vi "Update Field for Spartan 5.0.vi"(8 "error in (no error)":errorcluster, 10 "Old Field Record":T1={"ixField"=0, "iSequenceOrder"=0, "sxFieldId"="", "sxSequenceId"="", "sDisplayName"="", "sValue"="", "sUnits"="", "nDataType"=enum."timestamp", "nNextItem"=enum."Reset", "fSystem"=FALSE, "fSystemValue"=FALSE, "fRequired"=FALSE, "fSetAtTest"=FALSE, "fTestField"=FALSE, "fDeleted"=FALSE, "fIndexed"=FALSE, "fFreeList"=FALSE}) -> (0 "error out":errorcluster, 2 "New Field Record":T1={"ixField"=0, "iSequenceOrder"=0, "sxFieldId"="", "sxSequenceId"="", "sDisplayName"="", "sValue"="", "sUnits"="", "nDataType"=enum."timestamp", "nNextItem"=enum."Reset", "fSystem"=FALSE, "fSystemValue"=FALSE, "fRequired"=FALSE, "fSetAtTest"=FALSE, "fTestField"=FALSE, "fDeleted"=FALSE, "fIndexed"=FALSE, "fFreeList"=FALSE})   [LabVIEW 2011]
uses:
  Field Record.ctl
  Field DataTypes.ctl
  Field NextItem.ctl
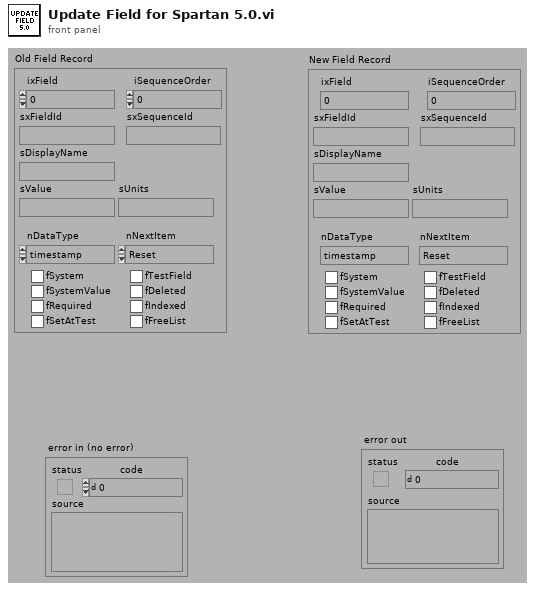
[diagram p1: front panel]
types:
  T1 = typedef "Field Record.ctl" = cluster{"ixField":i32, "iSequenceOrder":i32, "sxFieldId":string, "sxSequenceId":string, "sDisplayName":string, "sValue":string, "sUnits":string, "nDataType":T2, "nNextItem":T3, "fSystem":bool, "fSystemValue":bool, "fRequired":bool, "fSetAtTest":bool, "fTestField":bool, "fDeleted":bool, "fIndexed":bool, "fFreeList":bool}
  T2 = typedef "Field DataTypes.ctl" = enum32{"text", "numeric", "list", "timestamp", "boolean"}
  T3 = typedef "Field NextItem.ctl" = enum32{"Reset", "Retain", "Auto-Increment"}
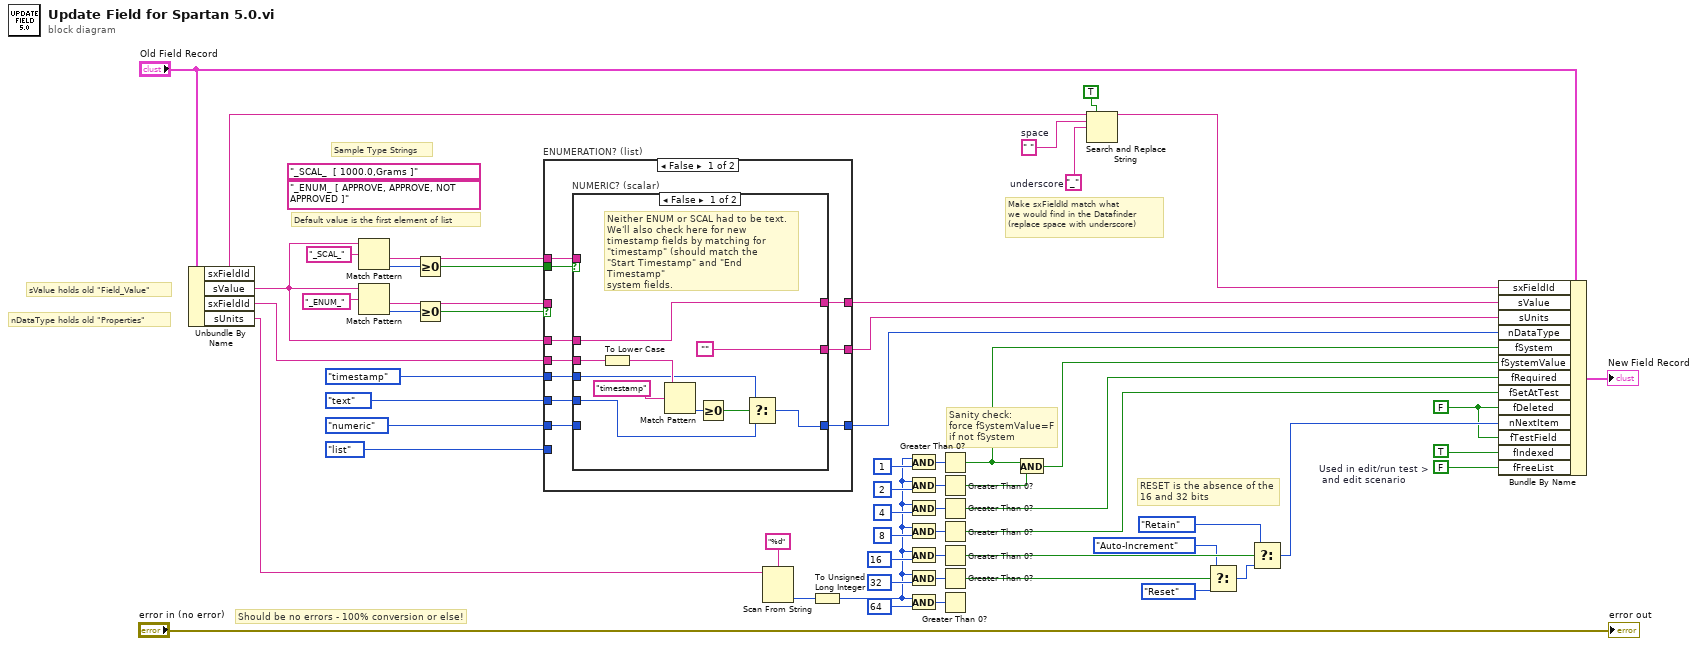
[diagram p0: block diagram]
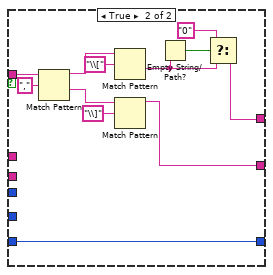
[diagram p2: hidden frame]
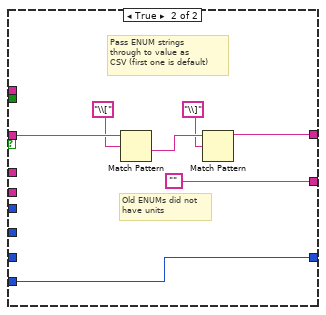
[diagram p3: hidden frame]
diagram:
  w6 = FALSE  # Used in edit/run test >  and edit scenario
  w9 = "_"  # underscore
  w10 = " "  # space
  (unwired) "_ENUM_ [ APPROVE, APPROVE, NOT APPROVED ]" ("Name")
  (unwired) "_SCAL_  [ 1000.0,Grams ]" ("Name")
  w1 = FALSE
  # "Sanity check:\nforce fSystemValue=F\nif not fSystem"
  # "Make sxFieldId match what\nwe would find in the Datafinder\n(replace space with underscore)"
  # "RESET is the absence of the \n16 and 32 bits"
  # "Default value is the first element of list"
  # "Sample Type Strings"
  # "sValue holds old \"Field_Value\""
  # "nDataType holds old \"Properties\""
  # "Should be no errors - 100% conversion or else!"
  n1 = Unbundle By Name("Old Field Record") -> ("sxFieldId"=w7:string, "sValue"=w40:string, "sxFieldId"=w39:string, "sUnits"=w17:string)
  n2 = Match Pattern(string=w40, regular expression="_SCAL_" ("search string/char (-)")) -> (after substring=w41:string, offset past match=w45:i32)  [unwired: 3 out]
  n3 = Match Pattern(string=w40, regular expression="_ENUM_" ("search string/char (-)")) -> (after substring=w42:string, offset past match=w43:i32)  [unwired: 3 out]
  n4 = Greater Or Equal To 0?(x=w45) -> (x >= 0?=w54:bool)
  n5 = Greater Or Equal To 0?(x=w43) -> (x >= 0?=w55:bool)
  n6 = case "ENUMERATION? (list)" shown="False" w55 {
    tunnel: [w61 ""] -> w48
    tunnel: [w68 w97] -> w49
    tunnel: w54 -> [w67 _]
    tunnel: Field_DataTypes."list" ("Field DataType") -> [_ w97]
    tunnel: Field_DataTypes."numeric" ("Field DataType") -> [w66 _]
    tunnel: Field_DataTypes."text" ("Field DataType") -> [w65 _]
    tunnel: Field_DataTypes."timestamp" ("Field DataType") -> [w64 _]
    tunnel: [w60 w92] -> w47
    tunnel: w42 -> [_ w96]
    tunnel: w41 -> [w63 _]
    tunnel: w40 -> [w62 _]
    tunnel: w39 -> [w59 _]
    frame False {
      n7 = case "NUMERIC? (scalar)" shown="False" w67 {
        tunnel: [w69 w90] -> w68
        tunnel: w66 -> [_ w90]
        tunnel: w65 -> [w70 _]
        tunnel: w64 -> [w71 _]
        tunnel: w63 -> [_ w84]
        tunnel: w62 -> [w77 _]
        tunnel: ["" w83] -> w61
        tunnel: [w77 w80] -> w60
        tunnel: w59 -> [w76 _]
        frame False {
          # "Neither ENUM or SCAL had to be text.\nWe'll also check here for new\ntimestamp fields by matching for\n\"timestamp\" (should match the\n\"Start Timestamp\" and \"End Timestamp\"\nsystem fields."
          n8 = To Lower Case(string=w76) -> (all lower case string=w75:string)
          n9 = Match Pattern(string=w75, regular expression="timestamp") -> (offset past match=w73:i32)  [unwired: 4 out]
          n10 = Greater Or Equal To 0?(x=w73) -> (x >= 0?=w72:bool)
          n11 = Select(t=w71, s=w72, f=w70) -> (s? t:f=w69:T2)
        }
        frame True {
          n12 = Match Pattern(string=w84, regular expression=",") -> (before substring=w87:string, after substring=w85:string)  [unwired: 3 out]
          n13 = Match Pattern(string=w87, regular expression="\\[") -> (after substring=w81:string)  [unwired: 4 out]
          n14 = Match Pattern(string=w85, regular expression="\\]") -> (before substring=w83:string)  [unwired: 4 out]
          n15 = Empty String/Path?(string/path=w81) -> (empty?=w82:bool)
          n16 = Select(t="0" ("regular expression"), s=w82, f=w81) -> (s? t:f=w80:string)
        }
      }
    }
    frame True {
      # "Old ENUMs did not\nhave units"
      # "Pass ENUM strings\nthrough to value as\nCSV (first one is default)"
      n17 = Match Pattern(string=w96, regular expression="\\[") -> (after substring=w94:string)  [unwired: 4 out]
      n18 = Match Pattern(string=w94, regular expression="\\]") -> (before substring=w92:string)  [unwired: 4 out]
    }
  }
  n19 = Scan From String(format string="%d", input string=w17) -> (output 1=w15:i32)  [unwired: 2 in, 4 out]
  n20 = To Unsigned Long Integer(number=w15) -> (unsigned 32bit integer=w21:u32)
  n21 = And(x=w21, y=u32 1) -> (x .and. y?=w37:u32)
  n22 = And(x=w21, y=u32 2) -> (x .and. y?=w36:u32)
  n23 = And(x=w21, y=u32 4) -> (x .and. y?=w33:u32)
  n24 = And(x=w21, y=u32 8) -> (x .and. y?=w22:u32)
  n25 = And(x=w21, y=u32 16) -> (x .and. y?=w29:u32)
  n26 = And(x=w21, y=u32 32) -> (x .and. y?=w28:u32)
  n27 = And(x=w21, y=u32 64) -> (x .and. y?=w32:u32)
  n28 = Greater Than 0?(x=w37) -> (x > 0?=w4:bool)
  n29 = Greater Than 0?(x=w36) -> (x > 0?=w3:bool)
  n30 = Greater Than 0?(x=w33) -> (x > 0?=w19:bool)
  n31 = Greater Than 0?(x=w22) -> (x > 0?=w18:bool)
  n32 = Greater Than 0?(x=w29) -> (x > 0?=w26:bool)
  n33 = Greater Than 0?(x=w28) -> (x > 0?=w25:bool)
  n34 = Greater Than 0?(x=w32) -> ()  [unwired: 1 out]
  n35 = And(x=w4, y=w3) -> (x .and. y?=w2:bool)
  n36 = Search and Replace String(replace all?=TRUE, input string=w7, search string=w10, replace string=w9) -> (result string=w8:string)  [unwired: 1 in, 6 out]
  n37 = Select(t=Field_NextItem."Auto-Increment" ("nNextItem"), s=w25, f=Field_NextItem."Reset" ("nNextItem")) -> (s? t:f=w24:T3)
  n38 = Select(t=Field_NextItem."Retain" ("nNextItem"), s=w26, f=w24) -> (s? t:f=w20:T3)
  n39 = Bundle By Name(cluster="Old Field Record", "sxFieldId"=w8, "sValue"=w47, "sUnits"=w48, "nDataType"=w49, "fSystem"=w4, "fSystemValue"=w2, "fRequired"=w19, "fSetAtTest"=w18, "fDeleted"=w1, "nNextItem"=w20, "fTestField"=w1, "fIndexed"=TRUE, "fFreeList"=w6) -> (→"New Field Record":T1)
  "error out" <- "error in (no error)"
